vi "Read Iteration.vi"(8 "error in (no error)":errorcluster, 11 "Stats_DBL_CIF_U in":refnum<class "Stats_DBL_CIF_U.lvclass">) -> (0 "error out":errorcluster, 2 "Iteration":u32, 3 "Stats_DBL_CIF_U out":refnum<class "Stats_DBL_CIF_U.lvclass">)   [LabVIEW 2021, in "Stats_CIF_U.lvlib" / "Stats_DBL_CIF_U.lvclass"]
uses:
  Stats_DBL_CIF_U.lvclass
  Stats_DBL_CIF_U.lvclass/Stats_DBL_CIF_U.ctl
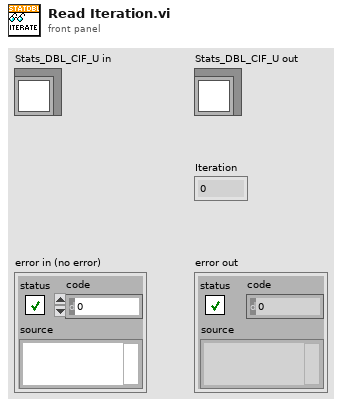
[diagram p1: front panel]
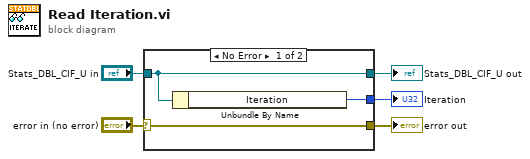
[diagram p0: block diagram]
diagram:
  n1 = case shown="No Error" "error in (no error)" {
    selector: "error in (no error)" -> [w8 w9]
    tunnel: [w8 w9] -> w4
    tunnel: [w7 w10] -> w2
    tunnel: "Stats_DBL_CIF_U in" -> [w7 w10]
    tunnel: [w6 _] -> w1
    frame No Error {
      n2 = Unbundle By Name(w7) -> ("Iteration"=w6:u32)
    }
    frame Error {
    }
  }
  "error out" <- w4
  "Stats_DBL_CIF_U out" <- w2
  "Iteration" <- w1
